vi "Test_4110.vi"() -> ()   [LabVIEW 2015]
panel:
  in  "Source:Output Enabled":bool
  in  "Stop":bool
  out "Compliance/Limit Reached 2":bool caption="Compliance/Limit Reached"
  out "Current Measurement 2":dbl caption="Current Measurement"
  out "Voltage Measurement 2":dbl caption="Voltage Measurement" format="%#_3g"
  in  "Channel Name 2":string="2"
  in  "Voltage Level 2":dbl=-15.0 caption="Voltage Level" format="%#.3p"
  in  "Source Delay (Sec)":dbl=0.1 format="%.3p"
  out "Voltage Measurement":dbl format="%#_3g"
  out "Current Measurement":dbl
  out "Compliance/Limit Reached":bool
  in  "Current Limit Range":dbl=1.0 format="%.3p"
  in  "Voltage Level Range":dbl=20.0 format="%.5p"
  in  "Current Limit":dbl=0.5 format="%.3p"
  in  "Voltage Level":dbl=15.0 format="%#.3p"
  in  "Channel Name":string="1" caption="Channel Name 1"
  in  "Resource Name":refnum<k15>="PXI1Slot6"
  # "V"
  # "V"
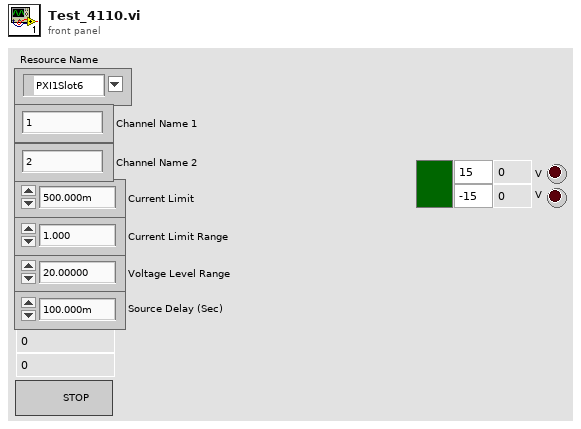
[diagram p1: front panel]
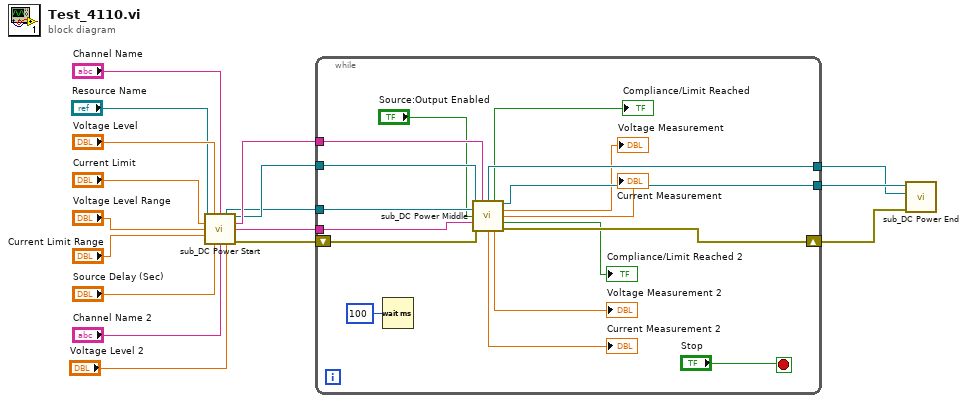
[diagram p0: block diagram]
diagram:
  n1 = call "sub_DC Power Start.vi"("IVI引用句柄输入"="Resource Name", "Voltage Level"="Voltage Level", "Channel Name"="Channel Name", "Current Limit"="Current Limit", "Voltage Level Range"="Voltage Level Range", "Current Limit Range"="Current Limit Range", "Source Delay (Sec)"="Source Delay (Sec)", "Channel Name 2"="Channel Name 2", "Voltage Level 2"="Voltage Level 2") -> ("instrument handle out"=w6:refnum<k15>, "IVI引用句柄输出"=w14:refnum<k15>, "Channel Name 4"=w15:string, "Channel Name 3"=w8:string, "错误输出"=w5:errorcluster)  [unwired: 2 in]
  n2 = while {
    tunnel: w15 -> [w34]
    tunnel: w8 -> [w33]
    tunnel: [w32] -> w7
    shift-right: [w31] -> w4
    shift-left: w5 -> [w27]
    tunnel: w6 -> [w26]
    tunnel: w14 -> [w28]
    tunnel: [w29] -> w16
    stop <- "Stop" stop-if-true
    n3 = Wait (ms)(milliseconds to wait=u32 100 ("等待时间（毫秒）")) -> ()  [unwired: 1 out]
    n4 = call "sub_DC Power Middle.vi"("IVI引用句柄输入"=w28, "Channel Name 4"=w34, "instrument handle out"=w26, "Source:Output Enabled"="Source:Output Enabled", "Channel Name 3"=w33, "错误输入（无错误）"=w27) -> ("instrument handle out 3"=w32:refnum<k15>, "Compliance/Limit Reached"=→"Compliance/Limit Reached":bool, "IVI引用句柄输出"=w29:refnum<k15>, "Voltage Measurement"=→"Voltage Measurement":dbl, "Current Measurement"=→"Current Measurement":dbl, "Compliance/Limit Reached 2"=→"Compliance/Limit Reached 2":bool, "Current Measurement 2"=→"Current Measurement 2":dbl, "Voltage Measurement 2"=→"Voltage Measurement 2":dbl, "错误输出"=w31:errorcluster)  [unwired: 1 in]
  }
  n5 = call "sub_DC Power End.vi"("错误输入（无错误）"=w4, "instrument handle out"=w7, "IVI引用句柄输入"=w16) -> ()  [unwired: 9 in]
